vi "wait.vi"(0 "HGF_NextMultiple":refnum<class "HGF_NextMultiple.lvclass">, 3 "msTimeout (-1)":i32=-1, 5 "error in (no error)":errorcluster, 9 "ignore previous (F)":bool) -> (14 "dup HGF_NextMultiple":refnum<class "HGF_NextMultiple.lvclass">, 16 "Object":refnum<class>, 17 "timed out":bool, 19 "error out":errorcluster)   [LabVIEW 2014, in "HGF_BaseClasses.lvlib" / "HGF_NextMultiple.lvclass"]
doc: "Use this VI to wait on next ms multiple of timeout value."
uses:
  HGF_NextMultiple.lvclass
  HGF_Event/HGF_Event.lvclass
  HGF_Timing/HGF_Timing.lvclass
  HGF_Auxiliary/HGF_Auxiliary.lvlib
  HGF_Auxiliary/Severity.ctl
  HGF_Auxiliary/ErrorCode.ctl
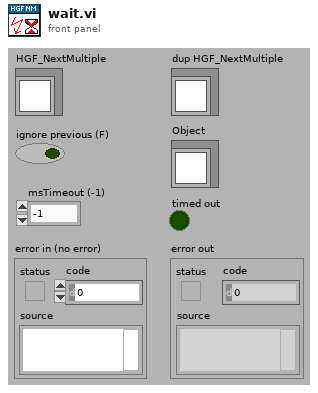
[diagram p1: front panel]
types:
  T1 = typedef "HGF_Auxiliary.lvlib/ErrorCode.ctl" = enum32{"No error", "Function not supported.", "This VI is for friends only.", "Reference object aready exisits.", "Parameter out of range.", "Not a rendezvous.", "Invalid notifier reference.", "Invalid queue reference.", "Self-Test not supported.", "Reset not supported.", "IDN query not supported.", "Error query not supported.", "Incorrect addressee.", "Object already exists.", "No class name specified", "Driver not supported", "Attribute is not writable"}
  T2 = typedef "HGF_Auxiliary.lvlib/Severity.ctl" = enum16{"Info", "Warning", "Fault", "Error", "Fatal"}
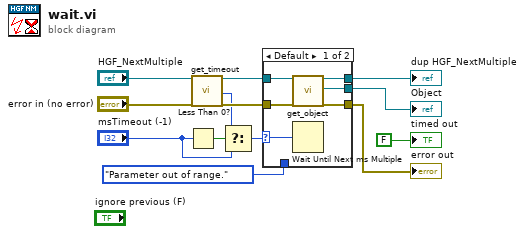
[diagram p0: block diagram]
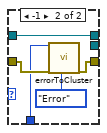
[diagram p2: hidden frame]
diagram:
  n1 = Less Than 0?(x="msTimeout (-1)") -> (x < 0?=w5:bool)
  n2 = call "get_timeout.vi"("HGF_Event.lvclass in"="HGF_NextMultiple", "error in (no error)"="error in (no error)") -> ("HGF_Event.lvclass out"=w8:refnum<class "HGF_NextMultiple.lvclass">, "timeout"=w3:i32, "error out"=w6:errorcluster)  [unwired: 15 out]
  n3 = Select(t=w3, s=w5, f="msTimeout (-1)") -> (s? t:f=w2:i32)
  n4 = case shown="Default" w2 {
    selector: w2 -> [w19 _]
    tunnel: [w16 w24] -> w12
    tunnel: [w14 _] -> w11
    tunnel: [w15 w22] -> w10
    tunnel: w8 -> [w18 w24]
    tunnel: w6 -> [w17 w23]
    tunnel: ErrorCode."Parameter out of range." ("error code") -> [_ w20]
    frame Default {
      n5 = call "get_object.vi"("HGF_Timing.lvclass"=w18, "error in (no error)"=w17) -> ("dup HGF_Timing"=w16:refnum<class "HGF_NextMultiple.lvclass">, "object"=w14:refnum<class>, "error out"=w15:errorcluster)  [unwired: 15 out]
      n6 = Wait Until Next ms Multiple(millisecond multiple=w19) -> ()  [unwired: 1 out]
    }
    frame -1 {
      n7 = call "errorToCluster.vi"("error code"=w20, "error in (no error)"=w23, "severity (Error)"=Severity."Error") -> ("error out"=w22:errorcluster)  [unwired: 2 in, 14 out]
    }
  }
  "error out" <- w10
  "dup HGF_NextMultiple" <- w12
  "Object" <- w11
  "timed out" <- FALSE ("timed out")
